vi "subExtractDependentExternalLib.vi"(10 "Owning lib name":string, 11 "Path":path) -> (3 "External lib":path)   [LabVIEW 2019, in "SolutionBuilder.lvlib" / "SolutionBuilder.lvclass"]
uses:
  SolutionBuilder.lvclass
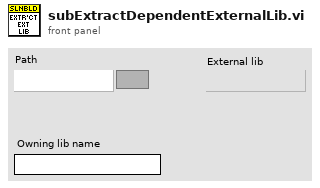
[diagram p1: front panel]
types:
  T1 = typedef "SolutionBuilder.lvlib/SolutionBuilder.lvclass/NamePathMap.ctl" = map{string, path}
  T2 = cluster{"count":i32, "name":string, "path":path}[]
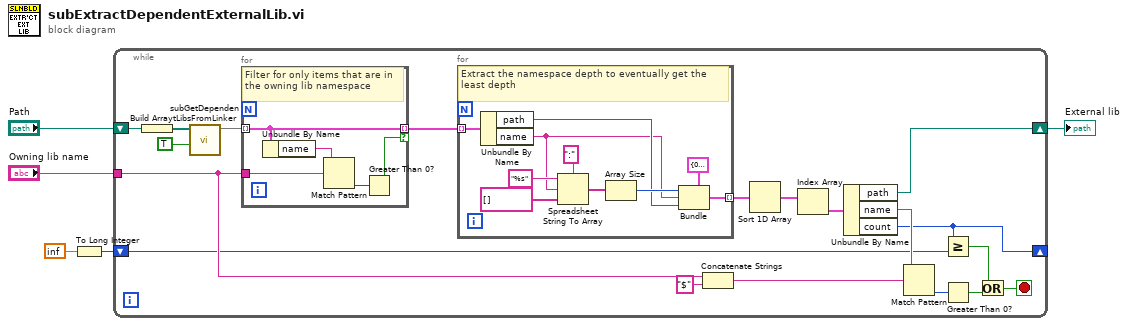
[diagram p0: block diagram]
diagram:
  n1 = To Long Integer(number=inf) -> (32bit integer=w2:i32)
  n2 = while {
    tunnel: "Owning lib name" -> [w16]
    shift-right: [w11] -> w1
    shift-left: "Path" -> [w23]
    shift-right: [w10] -> _
    shift-left: w2 -> [w9]
    stop <- w6 stop-if-true
    n3 = Build Array(w23) -> (w22:path[])
    n4 = call "subGetDependentLibsFromLinker.vi"("All?"=TRUE, "Paths"=w22) -> ("Dependency libs"=w21:T1)  [unwired: 8 in, 1 out]
    n5 = for {
      tunnel: w21 -> [w36] mode=indexing
      tunnel: w16 -> [w38]
      tunnel: [w36] -> w20 mode=indexing if=w35
      # "Filter for only items that are in the owning lib namespace"
      n6 = Unbundle By Name(w36) -> ("name"=w39:string)
      n7 = Match Pattern(string=w39, regular expression=w38) -> (offset past match=w37:i32)  [unwired: 1 in, 3 out]
      n8 = Greater Than 0?(x=w37) -> (x > 0?=w35:bool)
    }
    n9 = for {
      tunnel: w20 -> [w34] mode=indexing
      tunnel: [w27] -> w19 mode=indexing
      # "Extract the namespace depth to eventually get the least depth"
      n10 = Unbundle By Name(w34) -> ("path"=w28:path, "name"=w26:string)
      n11 = Spreadsheet String To Array(delimiter (Tab)=":", format string="%s", spreadsheet string=w26, array type (2D Dbl)=string[] []) -> (array=w30:string[])
      n12 = Array Size(array=w30) -> (size(s)=w29:i32)
      n13 = Bundle(cluster=cluster{"count":i32, "name":string, "path":path} {"count"=0, "name"="", "path"=path ""}, "count"=w29, "name"=w26, "path"=w28) -> (w27:cluster{"count":i32, "name":string, "path":path})
    }
    n14 = Concatenate Strings(w16, "$" ("string")) -> (w13:string)
    n15 = Sort 1D Array(array=w19) -> (sorted array=w18:T2)
    n16 = Index Array(array=w18) -> (element=w17:cluster{"count":i32, "name":string, "path":path})  [unwired: 1 in]
    n17 = Unbundle By Name(w17) -> ("path"=w11:path, "name"=w14:string, "count"=w10:i32)
    n18 = Match Pattern(string=w14, regular expression=w13) -> (offset past match=w12:i32)  [unwired: 1 in, 3 out]
    n19 = Greater Or Equal?(x=w10, y=w9) -> (x >= y?=w8:bool)
    n20 = Greater Than 0?(x=w12) -> (x > 0?=w7:bool)
    n21 = Or(x=w8, y=w7) -> (x .or. y?=w6:bool)
  }
  "External lib" <- w1
